vi "myRIO_BRig_FPGA_v3,51.vi"() -> ()   [LabVIEW 2014]
uses:
  <vilib>/rvi/Emulation/niFpgaGetClockAttributes.vi
  <vilib>/rvi/Emulation/niFpgaSctlEmulationGetInTimedLoop.vi
  <vilib>/rvi/Emulation/niFpgaEmulationReportErrorSimple.vi
  <vilib>/rvi/eio/common/nirviEmuTemplateMethod_errors.vi
  <vilib>/rvi/Emulation/niFpgaCriticalErrorInLSC.vi
  <vilib>/eio/EIONode/EIONode.xnode
panel:
  out "output_audioValue_R":i16
  out "output_audioValue_L":i16
  out "count_timeTrial":u32
  in  "timeTrial":bool
  in  "k1__counter_per_ms":u16=100 min=100 max=40000 step=1
  in  "laser_Nshutter":u32=100
  in  "AnaOut_0":u16
  in  "laser_Nvalley":u32=100
  in  "laser_Npeak":u32=100
  in  "laserledMTrig":bool
  in  "laser_selWro_Ntotal":u32=100
  in  "laser_selWro_NDelay":u32
  in  "laser_selRew_Ntotal":u32=100
  in  "laser_selRew_Ndelay":u32
  in  "laserResponse_reward_LED":bool
  in  "laserResponse_wrong_LED":bool
  out "SelectWrong":bool
  out "SelectReward":bool
  in  "laserResponse_wrong":bool
  in  "laserResponse_reward":bool
  in  "Left(F)_or_Right(T)":bool
  in  "ignoreWrong":bool
  in  "SelectionState":bool
  in  "laserMTrig":bool
  in  "FPGA_Stop":bool
  in  "audioTrigger_L":bool
  in  "audioTrigger_R":bool
  in  "audioFreq_L_kHz":u8=14 min=1 max=14 step=1
  in  "audioAmp_L":u16=1 min=1 max=32767 step=1
  in  "audioFreq_R_kHz":u8=14 min=1 max=14 step=1
  in  "audioAmp_R":u16=1 min=1 max=32767 step=1
  in  "A3_SL":bool
  in  "A1_SR":bool
  in  "Counts_Reset":bool
  out "A4_LickR":u32
  out "A2_LickL":u32
  in  "A6_Act":bool
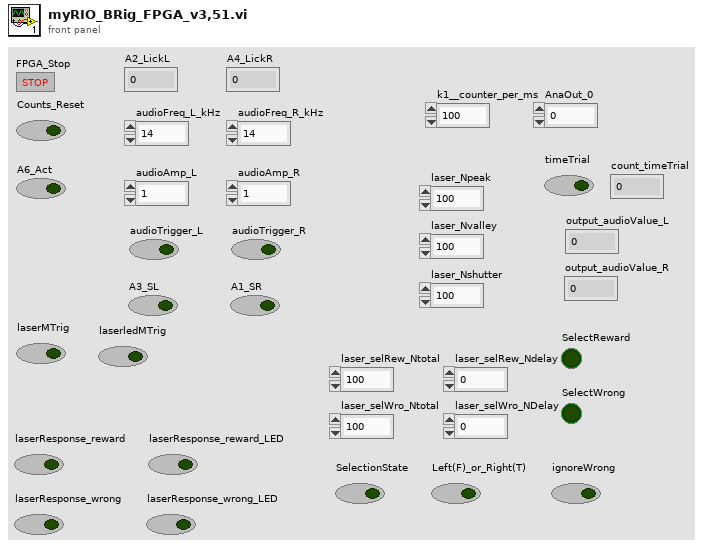
[diagram p1: front panel]
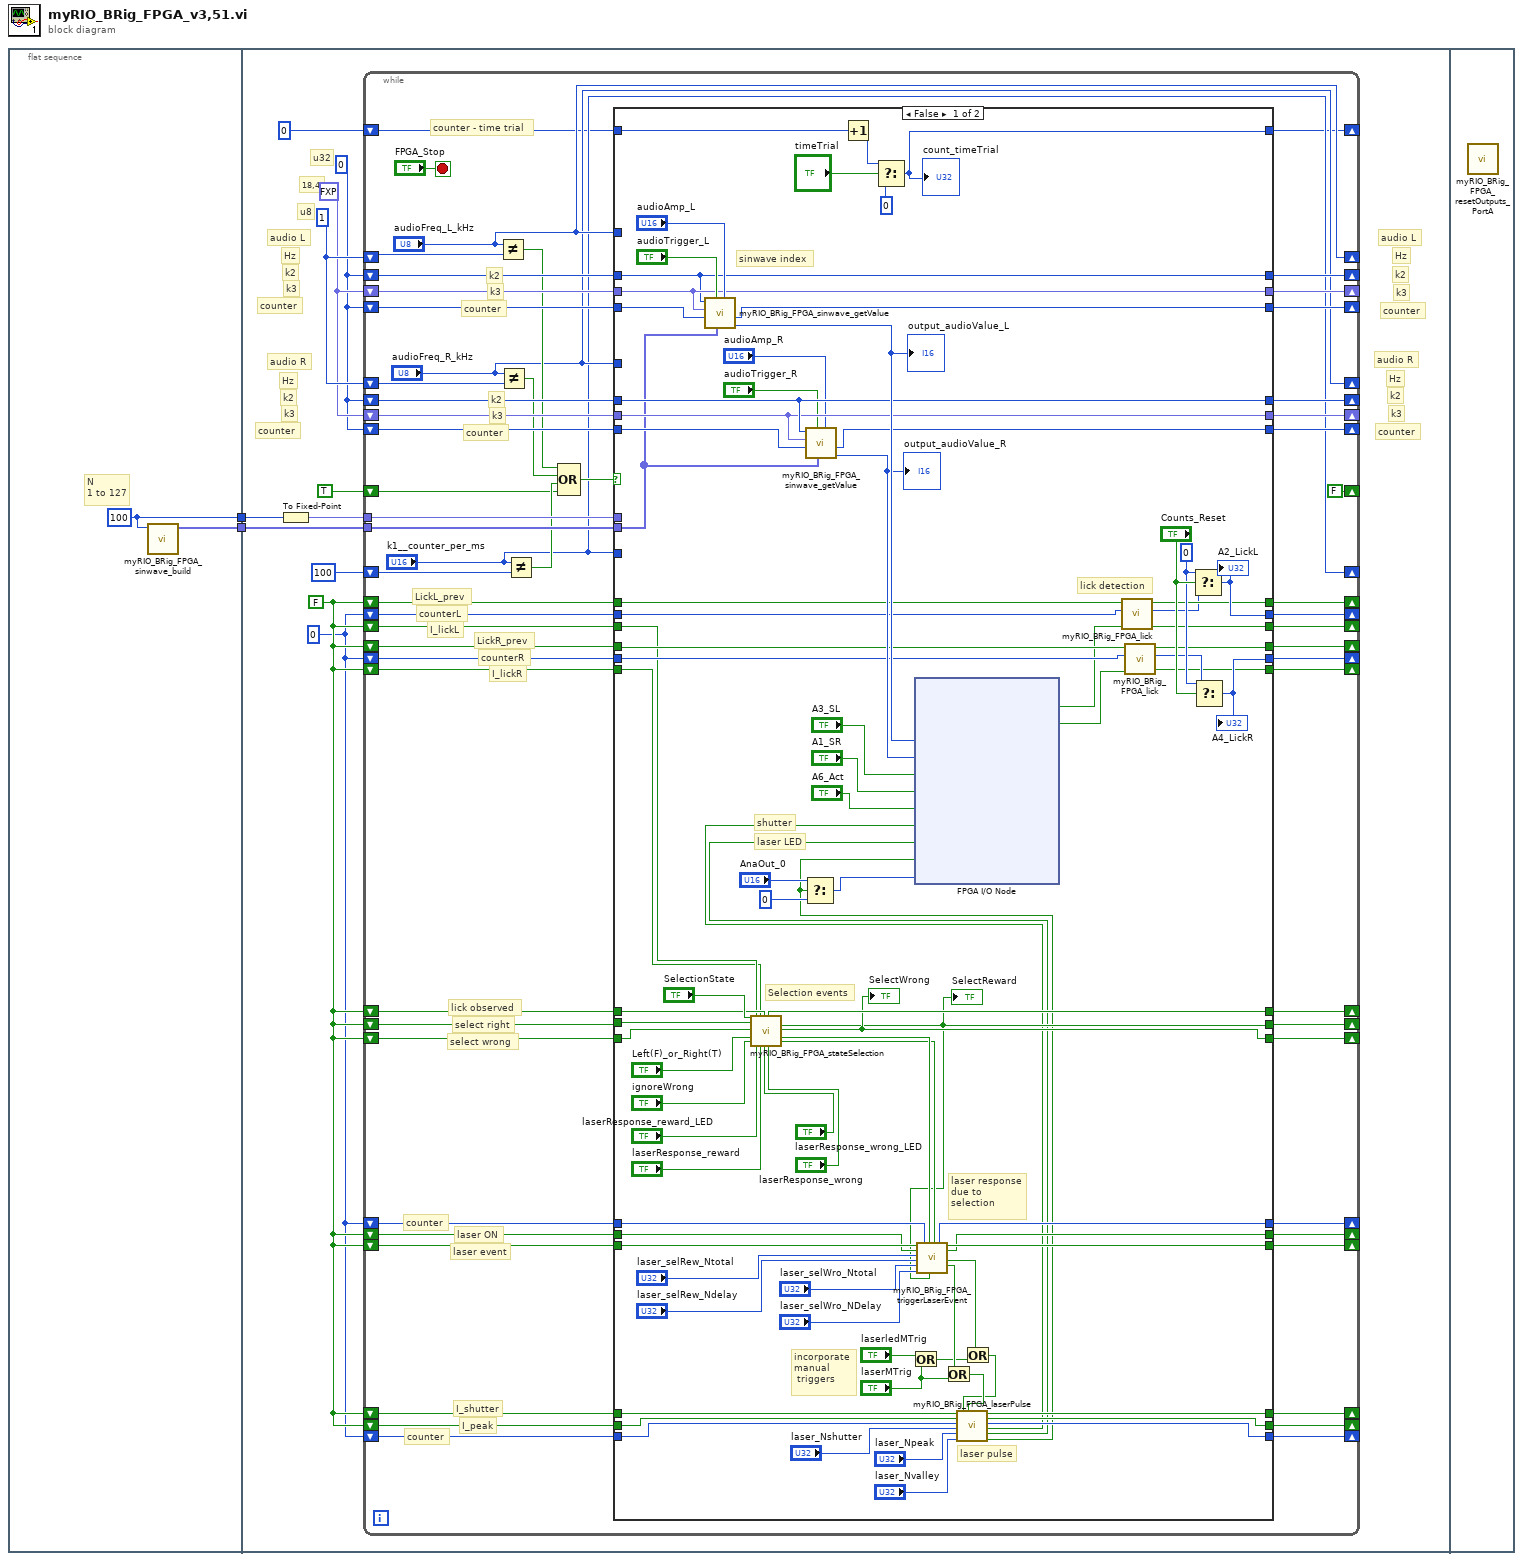
[diagram p0: block diagram]
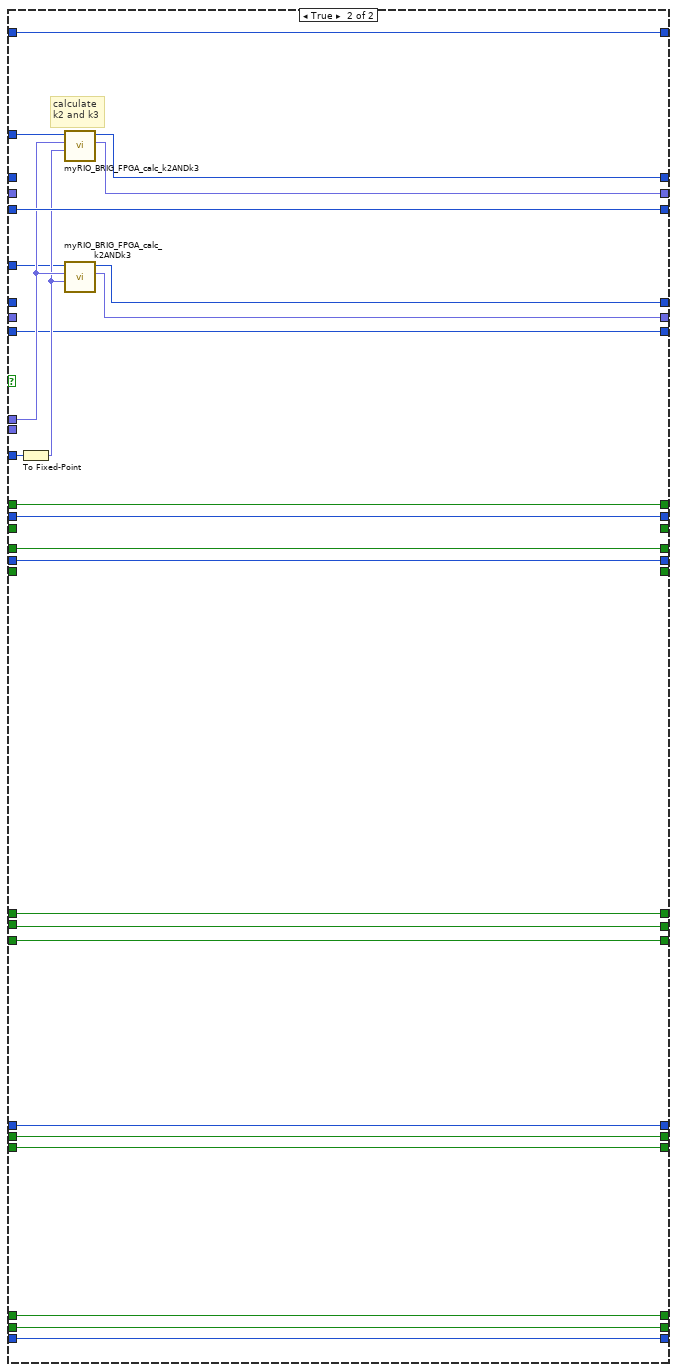
[diagram p2: hidden frame]
diagram:
  n1 = flat-sequence {
    tunnel: [w4] -> w2
    tunnel: [w3] -> w1
    tunnel: w2 -> [w15]
    tunnel: w1 -> [w14]
    frame #0 {
      w3 = 100 ("dimension size")
      # "N\n1 to 127"
      n2 = call "myRIO_BRig_FPGA_sinwave_build.vi"("input_Npts"=w3) -> ("output_array_sin"=w4:fxp<+/-,16,2>[])  [unwired: 10 in]
    }
    frame #1 {
      w6 = u32 0
      w7 = FALSE
      w10 = u32 0
      w11 = fxp<+,18,4> 0.0
      w12 = u8 1
      # "counter"
      # "k3"
      # "k2"
      # "counter"
      # "k3"
      # "k2"
      # "counter"
      # "counter"
      # "u32"
      # "k3"
      # "k2"
      # "k3"
      # "18,4"
      # "u8"
      # "Hz"
      # "Hz"
      # "audio R"
      # "audio L"
      # "Hz"
      # "k2"
      # "Hz"
      # "audio R"
      # "audio L"
      n3 = To Fixed-Point(number=w14) -> (fixed-point=w13:fxp<+,7,7>)  [unwired: 1 in]
      n4 = while {
        shift-right: ["audioFreq_L_kHz"] -> _
        shift-left: w12 -> [w74]
        shift-right: [w68] -> _
        shift-left: w10 -> [w72]
        shift-right: ["audioFreq_R_kHz"] -> _
        shift-left: w12 -> [w64]
        tunnel: w15 -> [w71]
        tunnel: w13 -> [w70]
        shift-right: [w67] -> _
        shift-left: w11 -> [w69]
        shift-right: [w65] -> _
        shift-left: w10 -> [w66]
        shift-right: [w62] -> _
        shift-left: w10 -> [w63]
        shift-right: [w60] -> _
        shift-left: w11 -> [w61]
        shift-right: [w58] -> _
        shift-left: w10 -> [w59]
        shift-right: ["k1__counter_per_ms"] -> _
        shift-left: u16 100 ("y") -> [w57]
        shift-right: [FALSE] -> _
        shift-left: TRUE -> [w52]
        shift-right: [w45] -> _
        shift-left: w7 -> [w47]
        shift-right: [w44] -> _
        shift-left: w7 -> [w46]
        shift-right: [w42] -> _
        shift-left: w6 -> [w43]
        shift-right: [w40] -> _
        shift-left: w6 -> [w41]
        shift-right: [w38] -> _
        shift-left: w7 -> [w39]
        shift-right: [w35] -> _
        shift-left: w7 -> [w37]
        shift-right: [w34] -> _
        shift-left: w7 -> [w36]
        shift-right: [w31] -> _
        shift-left: w7 -> [w30]
        shift-right: [w32] -> _
        shift-left: w7 -> [w33]
        shift-right: [w28] -> _
        shift-left: w6 -> [w29]
        shift-right: [w24] -> _
        shift-left: w7 -> [w27]
        shift-right: [w23] -> _
        shift-left: w7 -> [w26]
        shift-right: [w22] -> _
        shift-left: w6 -> [w25]
        shift-right: [w20] -> _
        shift-left: w7 -> [w21]
        shift-right: [w18] -> _
        shift-left: w7 -> [w19]
        shift-right: [w16] -> _
        shift-left: u32 0 -> [w17]
        stop <- "FPGA_Stop" stop-if-true
        # "counter"
        # "k3"
        # "k2"
        # "counter"
        # "k3"
        # "k2"
        # "counter - time trial"
        # "counter"
        # "counter"
        # "I_lickR"
        # "counterR"
        # "LickR_prev"
        # "I_lickL"
        # "counterL"
        # "LickL_prev"
        # "I_shutter"
        # "I_peak"
        # "laser ON"
        # "laser event"
        # "select wrong"
        # "select right"
        # "lick observed"
        n5 = Not Equal?(x="audioFreq_L_kHz", y=w74) -> (x != y?=w56:bool)
        n6 = Not Equal?(x="audioFreq_R_kHz", y=w64) -> (x != y?=w55:bool)
        n7 = Not Equal?(x="k1__counter_per_ms", y=w57) -> (x != y?=w53:bool)
        n8 = Compound Arithmetic op=OR(w56, w55, w53, w52) -> (w54:bool)
        n9 = case shown="False" w54 {
          tunnel: w72 -> [w124 _]
          tunnel: "audioFreq_L_kHz" -> [_ w186]
          tunnel: w71 -> [w116 _]
          tunnel: w70 -> [_ w182]
          tunnel: "k1__counter_per_ms" -> [_ w187]
          tunnel: w69 -> [w125 _]
          tunnel: [w124 w185] -> w68
          tunnel: [w125 w184] -> w67
          tunnel: w66 -> [w130 w183]
          tunnel: [w127 w183] -> w65
          tunnel: w63 -> [w120 _]
          tunnel: [w120 w178] -> w62
          tunnel: w61 -> [w119 _]
          tunnel: [w119 w179] -> w60
          tunnel: w59 -> [w123 w177]
          tunnel: "audioFreq_R_kHz" -> [_ w180]
          tunnel: [w122 w177] -> w58
          tunnel: w47 -> [w111 w176]
          tunnel: w46 -> [w110 w175]
          tunnel: [w115 w176] -> w45
          tunnel: [w108 w175] -> w44
          tunnel: w43 -> [w112 w174]
          tunnel: [w162 w174] -> w42
          tunnel: w41 -> [w109 w173]
          tunnel: [w159 w173] -> w40
          tunnel: w39 -> [w152 w172]
          tunnel: [w151 w172] -> w38
          tunnel: w37 -> [w154 w171]
          tunnel: w36 -> [w153 w170]
          tunnel: [w99 w171] -> w35
          tunnel: [w144 w170] -> w34
          tunnel: w33 -> [w142 w169]
          tunnel: [w138 w169] -> w32
          tunnel: [w139 w168] -> w31
          tunnel: w30 -> [w143 w168]
          tunnel: w29 -> [w141 w167]
          tunnel: [w140 w167] -> w28
          tunnel: w27 -> [w93 w166]
          tunnel: w26 -> [w94 w165]
          tunnel: w25 -> [w95 w164]
          tunnel: [w96 w166] -> w24
          tunnel: [w97 w165] -> w23
          tunnel: [w98 w164] -> w22
          tunnel: w21 -> [w103 _]
          tunnel: [w114 _] -> w20
          tunnel: w19 -> [w102 _]
          tunnel: [w106 _] -> w18
          tunnel: w17 -> [w79 w163]
          tunnel: [w76 w163] -> w16
          frame False {
            w160 = u32 0 ("t")
            # "sinwave index"
            # "lick detection"
            # "laser pulse"
            # "incorporate\nmanual\n triggers"
            # "laser response\ndue to\nselection"
            # "Selection events"
            # "laser LED"
            # "shutter"
            n10 = call "myRIO_BRig_FPGA_sinwave_getValue.vi"("audioAmp"="audioAmp_L", "sinwave"=w116, "audioTrigger"="audioTrigger_L", "counter"=w130, "k3"=w125, "k2"=w124) -> ("output_audioValue"=w126:i16, "output_counter"=w127:u32)  [unwired: 4 in]
            "output_audioValue_L" <- w126
            n11 = call "myRIO_BRig_FPGA_stateSelection.vi"("I_selectionState"="SelectionState", "I_selectRight"=w154, "I_selectWrong"=w153, "I_Left(F)_or_Right(T)"="Left(F)_or_Right(T)", "I_ignoreWrong"="ignoreWrong", "I_lickL"=w103, "I_laserEvent_Reward"="laserResponse_reward_LED", "I_lickR"=w102, "I_laser_Reward"="laserResponse_reward", "I_lickObserved"=w152, "I_laserEvent_Wrong"="laserResponse_wrong_LED", "I_laser_Wrong"="laserResponse_wrong") -> ("output_I_lickObserved"=w151:bool, "output__I_selectRight"=w99:bool, "output__I_selectWrong"=w144:bool, "output_I_startLaserEvent"=w101:bool, "output_I_startLaser"=w100:bool)  [unwired: 11 in]
            "SelectWrong" <- w144
            "SelectReward" <- w99
            n12 = call "myRIO_BRig_FPGA_sinwave_getValue.vi"("audioAmp"="audioAmp_R", "sinwave"=w116, "audioTrigger"="audioTrigger_R", "counter"=w123, "k3"=w119, "k2"=w120) -> ("output_audioValue"=w121:i16, "output_counter"=w122:u32)  [unwired: 4 in]
            "output_audioValue_R" <- w121
            n13 = Increment(x=w79) -> (x+1=w78:u32)
            n14 = Select(t=w78, s="timeTrial", f=u32 0) -> (s? t:f=w76:u32)
            "count_timeTrial" <- w76
            n15 = Or(x="laserledMTrig", y="laserMTrig") -> (x .or. y?=w83:bool)
            n16 = call "myRIO_BRig_FPGA_triggerLaserEvent.vi"("I_laserEvent"=w143, "I_laser"=w142, "laser_selRew_Ntotal"="laser_selRew_Ntotal", "laser_selRew_Ndelay"="laser_selRew_Ndelay", "laser_selWro_Ntotal"="laser_selWro_Ntotal", "laser_selWro_NDelay"="laser_selWro_NDelay", "counter"=w141, "I_startLaserEvent"=w101, "selectReward"=w99, "I_startLaser"=w100) -> ("output_counter"=w140:u32, "output_I_laserEvent"=w139:bool, "output_I_laser"=w138:bool, "output_I_trigLaserEvent"=w85:bool, "output_I_trigLaser"=w84:bool)  [unwired: 5 in]
            n17 = Or(x=w84, y="laserMTrig") -> (x .or. y?=w81:bool)
            n18 = Or(x=w85, y=w83) -> (x .or. y?=w80:bool)
            n19 = call "myRIO_BRig_FPGA_laserPulse.vi"("I_shutter"=w93, "I_peak"=w94, "count"=w95, "laser_Nshutter"="laser_Nshutter", "laser_Npeak"="laser_Npeak", "laser_Nvalley"="laser_Nvalley", "I_laserEvent"=w80, "I_laser"=w81) -> ("output_I_shutter"=w96:bool, "output_I_peak"=w97:bool, "output_count"=w98:u32, "output_shutter"=w89:bool, "output_led"=w88:bool, "output_laser"=w87:bool)  [unwired: 6 in]
            n20 = Select(t="AnaOut_0", s=w87, f=u16 0) -> (s? t:f=w86:u16)
            n21 = xnode "FPGA I/O Node"("AudioOut/Left"=w126, "AudioOut/Right"=w121, "ConnectorA/DIO3"="A3_SL", "ConnectorA/DIO1"="A1_SR", "ConnectorA/DIO7"="A6_Act", "ConnectorA/DIO6"=w89, "ConnectorA/DIO14"=w88, "ConnectorA/DIO0"=w87, "ConnectorB/AO0"=w86) -> ("ConnectorA/DIO2"=w105:bool, "ConnectorA/DIO4"=w104:bool)  [unwired: 11 in, 11 out]
            n22 = call "myRIO_BRig_FPGA_lick.vi"("I_stateDetector_new"=w105, "counter"=w112, "I_stateDetector_prev"=w111) -> ("output_I_lick"=w114:bool, "output_counter"=w113:u32, "output_I_stateDetector_prev"=w115:bool)  [unwired: 6 in]
            n23 = call "myRIO_BRig_FPGA_lick.vi"("I_stateDetector_new"=w104, "counter"=w109, "I_stateDetector_prev"=w110) -> ("output_I_lick"=w106:bool, "output_counter"=w107:u32, "output_I_stateDetector_prev"=w108:bool)  [unwired: 6 in]
            n24 = Select(t=w160, s="Counts_Reset", f=w113) -> (s? t:f=w162:u32)
            "A2_LickL" <- w162
            n25 = Select(t=w160, s="Counts_Reset", f=w107) -> (s? t:f=w159:u32)
            "A4_LickR" <- w159
          }
          frame True {
            # "calculate\nk2 and k3"
            n26 = To Fixed-Point(number=w187) -> (fixed-point=w181:fxp<+,16,16>)  [unwired: 1 in]
            n27 = call "myRIO_BRIG_FPGA_calc_k2ANDk3.vi"("input_k1[count/ms]"=w181, "input_Npts"=w182, "input_freq[kHz]"=w186) -> ("output_k3"=w184:fxp<+,18,4>, "output_k2"=w185:u32)  [unwired: 7 in]
            n28 = call "myRIO_BRIG_FPGA_calc_k2ANDk3.vi"("input_k1[count/ms]"=w181, "input_Npts"=w182, "input_freq[kHz]"=w180) -> ("output_k3"=w179:fxp<+,18,4>, "output_k2"=w178:u32)  [unwired: 7 in]
          }
        }
      }
    }
    frame #2 {
      n29 = call "myRIO_BRig_FPGA_resetOutputs_PortA.vi"() -> ()  [unwired: 12 in]
    }
  }
